vi "sender.vi"() -> ()   [LabVIEW 2018]
uses:
  <vilib>/sound2/lvsound2.llb/Sound Data Format.ctl
  <vilib>/sound2/lvsound2.llb/Sampling Mode.ctl
  <vilib>/sound2/lvsound2.llb/Sound Input Read (DBL).vi
panel:
  in  "sound format":T1={"sample rate (S/s)"=22050.0, "number of channels"=2, "bits per sample"=16}
  in  "number of samples/ch":i32=100000
  in  "stop":bool
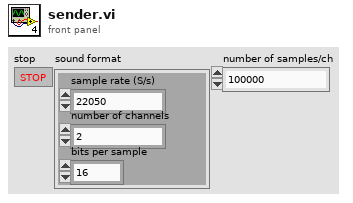
[diagram p1: front panel]
types:
  T1 = typedef "Sound Data Format.ctl" = cluster{"sample rate (S/s)":dbl, "number of channels":i32, "bits per sample":i32}
  T2 = typedef "Sampling Mode.ctl" = i32
  T3 = enum16{"Read", "Write", "ReadWrite", "BufferedRead", "BufferedReadWrite"}
  T4 = typedef "Sound Input Task ID.ctl" = u32
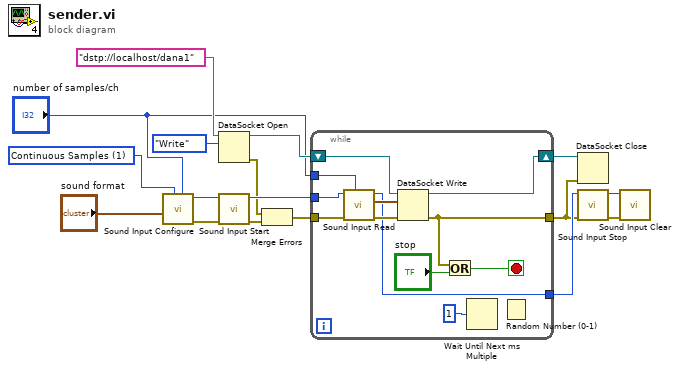
[diagram p0: block diagram]
diagram:
  w2 = T2 1 items=["Finite Samples", "Continuous Samples"] ("sample mode")
  n1 = call <vilib>:"Sound Input Configure.vi"("number of samples/ch"="number of samples/ch", "sample mode"=w2, "sound format"="sound format") -> ("error out"=w12:errorcluster, "task ID"=w13:T4)  [unwired: 7 in]
  n2 = DataSocket Open(10:T3."Write" ("mode"), 11:"dstp://localhost/dana1" ("URL")) -> (0:w4:errorcluster, 3:w16:refnum<k13>)  [unwired: 2 in]
  n3 = call <vilib>:"Sound Input Start.vi"("error in (no error)"=w12, "task ID"=w13) -> ("error out"=w5:errorcluster, "task ID out"=w11:T4)  [unwired: 8 in]
  n4 = Merge Errors(w4, w5) -> (w6:errorcluster)
  n5 = while {
    shift-right: [w28] -> w15
    shift-left: w16 -> [w29]
    tunnel: w11 -> [w24]
    tunnel: [w21] -> w7
    tunnel: w6 -> [w20]
    tunnel: [w19] -> w3
    tunnel: "number of samples/ch" -> [w18]
    stop <- w26 stop-if-true
    n6 = call-poly <vilib>:"Sound Input Read.vi"("number of samples/ch"=w18, "error in (no error)"=w20, "task ID"=w24) -> ("error out"=w22:errorcluster, "data"=w23:waveform(dbl)[], "task ID out"=w21:T4)  [unwired: 6 in]
    n7 = DataSocket Write(8:w22, 10:w23, 11:w29) -> (0:w19:errorcluster, 3:w28:refnum<k13>)  [unwired: 1 in, 1 out]
    n8 = Or(x=w19, y="stop") -> (x .or. y?=w26:bool)
    n9 = Wait Until Next ms Multiple(millisecond multiple=u32 1) -> ()  [unwired: 1 out]
    n10 = Random Number (0-1)() -> ()  [unwired: 1 out]
  }
  n11 = DataSocket Close(8:w3, 11:w15) -> ()  [unwired: 1 in, 2 out]
  n12 = call <vilib>:"Sound Input Stop.vi"("error in (no error)"=w3, "task ID"=w7) -> ("error out"=w10:errorcluster, "task ID out"=w9:T4)  [unwired: 8 in]
  n13 = call <vilib>:"Sound Input Clear.vi"("error in (no error)"=w10, "task ID"=w9) -> ()  [unwired: 9 in, 1 out]
